vi "Control Experiment.vi"() -> ()   [LabVIEW 2016, in "Transport.lvclass"]
uses:
  Transport.lvclass
  <userlib>/LevyLab/Krohn Hite 7008/typedefs/Shunt-Enum.ctl
  <userlib>/LevyLab/Krohn Hite 7008/typedefs/Gain-Enum.ctl
  <userlib>/LevyLab/Krohn Hite 7008/typedefs/KH_control_array.ctl
  <userlib>/LevyLab/Krohn Hite 7008/typedefs/KH_control.ctl
  <userlib>/LevyLab/Krohn Hite 7008/typedefs/Channel-Enum.ctl
  <userlib>/LevyLab/Krohn Hite 7008/typedefs/Input Configuration-Enum.ctl
  levylab_inst_pickering/lvsrc/SMOs/pickering/Typedefs/PickeringConfig-Cluster.ctl
  levylab_inst_pickering/lvsrc/SMOs/pickering/Typedefs/PickeringXConfig-Cluster.ctl
  levylab_inst_pickering/lvsrc/SMOs/pickering/Typedefs/PickeringYConfig-Cluster.ctl
  Control Experiment FGV-cluster.ctl
  ITX_Global.vi
  Channel Global.vi
  <userlib>/LevyLab/Krohn Hite 7008/KH7008.lvclass
  <vilib>/addons/_JKI.lib/Serialization/JSON/JKI JSON Serialization.lvlib
  levylab_inst_pickering/lvsrc/SMOs/pickering/pickering.lvclass
panel:
  in  "Create Output":bool
  in  "OK":bool
  in  "Tab Control":T1(tab)=enum."Pickering Configuration"
  in  "Pickering Buttons":enum32{"Pickering", "Not Pickering"}(radio)
  in  "description":string="graphene"
  in  "KH Configuration":enum16{"Ground", "Current", "Voltage", "Gate"}[](array[ring])=[enum."Current", enum."Current", enum."Ground", enum."Ground", enum."Ground", enum."Ground", enum."Ground", enum."Ground"]
  in  "KH Shunt Resistor":T2[](array[typedef])=[enum."50 Ohms", enum."50 Ohms", enum."50 Ohms", enum."50 Ohms", enum."50 Ohms", enum."50 Ohms", enum."50 Ohms", enum."50 Ohms"]
  in  "KH Gain":T3[](array[typedef])=[enum."10x", enum."10x", enum."10x", enum."10x", enum."10x", enum."10x", enum."10x", enum."10x"]
  in  "KH Ch":enum16{"1", "2", "3", "4", "5", "6", "7", "8"}[](array[ring])=[enum."1", enum."2", enum."3", enum."4", enum."5", enum."6", enum."7", enum."8"]
  in  "Electrode":T4(array[ring])=[enum."26", enum."26", enum."NC", enum."NC", enum."NC", enum."NC", enum."NC", enum."NC"]
  in  "Lockin Ch":enum16{"1", "2", "3", "4", "5", "6", "7", "8"}[](array[ring])=[enum."1", enum."2", enum."3", enum."4", enum."5", enum."6", enum."7", enum."8"]
  in  "Label":u16[](array[ring]) items=["", "I+", "I-", "V1+", "V1-", "V2+", "V2-", "V3+", "V3-", "V4+", "V4-", "Vsg", "Vbg"]
  in  "sample":string="SA01234"
  in  "device 2":string="20180713"
  in  "project (enum?)":string="graphene"
  in  "user (emum?)":string="patrick"
  in  "canvas":string="SA01234"
  in  "KH ALL Buttons":T5(radio)
  in  "Write Pickering Config":bool
  in  "Labels":u16[](array[ring]) items=["", "I+", "I-", "V1+", "V1-", "V2+", "V2-", "V3+", "V3-", "V4+", "V4-", "Vsg", "Vbg"]
  in  "Electrodes":T4(array[ring])
  in  "Y Channels":string[][](array[combo])=[["y1", "NC"], ["y2", "NC"], ["y3", ""], ["y4", ""], ["y5", ""], ["y6", ""], ["y7", ""], ["y8", ""], ["NC", ""], ["y7", ""], ["y6", ""]]
  in  "X Channels":string[](array[combo])=["x1", "x2", "x3", "x4", "x5", "x6", "x7", "x8", "x9", "x10", "x11", "x12"]
  out "X Channel Array":string[](array[string])
  out "Y Channel Array":string[][](array[string])
  in  "Read Pickering Config":bool
  out "device":string="SA01234SA01234.20180713"
  out "comments":string="SA01234SA01234.20180713\rgraphene\rpatrick\r2018-08-29T14:08:0929\r\rLockin1: 26\tI+\rLockin2: 26\tI-\rLockin3: NC\tV4-\rLockin4: NC\tV2+\rLockin5: NC\tV3+\rLockin6: NC\tV2-\rLockin7: NC\tV1+\rLockin8: NC\tV4+\r\n"
  out "folder":string="G:\\Team Drives\\LevyLabData\\graphene\\SA01234SA01234.20180713"
  out "filename":string="SA01234SA01234.20180713"
  out "JSON String":string="{\r\n    \"sample\":\"SA01234\",\r\n    \"canvas\":\"SA01234\",\r\n    \"date\":\"20180713\",\r\n    \"user\":\"patrick\",\r\n    \"project\":\"graphene\",\r\n    \"path\":\"G:\\\\Team Drives\\\\LevyLabData\\\\graphene\\\\SA01234SA01234.20180713\",\r\n    \"device\":\"SA01234SA01234.20180713\",\r\n    \"Channel Setting\":[\r\n        {\r\n            \"Channel\":\"Channel 1\",\r\n            \"Gain\":\"10x\",\r\n            \"Shunt Resistor\":\"50 Ohms\",\r\n            \"Input Config\":\"Differential\"\r\n        },\r\n        {\r\n            \"Channel\":\"Channel 2\",\r\n            \"Gain\":\"10x\",\r\n            \"Shunt Resistor\":\"50 Ohms\",\r\n            \"Input Config\":\"Differential\"\r\n        },\r\n        {\r\n            \"Channel\":\"Channel 3\",\r\n            \"Gain\":\"1x\",\r\n            \"Shunt Resistor\":\"Open\",\r\n            \"Input Config\":\"Ground\"\r\n        },\r\n        {\r\n            \"Channel\":\"Channel 4\",\r\n            \"Gain\":\"1x\",\r\n            \"Shunt Resistor\":\"Open\",\r\n            \"Input Config\":\"Ground\"\r\n        },\r\n        {\r\n            \"Channel\":\"Channel 5\",\r\n            \"Gain\":\"1x\",\r\n            \"Shunt Resistor\":\"Open\",\r\n            \"Input Config\":\"Ground\"\r\n        },\r\n        {\r\n            \"Channel\":\"Channel 6\",\r\n            \"Gain\":\"1x\",\r\n            \"Shunt Resistor\":\"Open\",\r\n            \"Input Config\":\"Ground\"\r\n        },\r\n        {\r\n            \"Channel\":\"Channel 7\",\r\n            \"Gain\":\"1x\",\r\n            \"Shunt Resistor\":\"Open\",\r\n            \"Input Config\":\"Ground\"\r\n        },\r\n        {\r\n            \"Channel\":\"Channel 8\",\r\n            \"Gain\":\"1x\",\r\n            \"Shunt Resistor\":\"Open\",\r\n            \"Input Config\":\"Ground\"\r\n        }\r\n    ],\r\n    \"All same as ch1?\":false,\r\n    \"Lockin Ch\":[\r\n        \"1\",\r\n        \"2\",\r\n        \"3\",\r\n        \"4\",\r\n        \"5\",\r\n        \"6\",\r\n        \"7\",\r\n        \"8\"\r\n    ],\r\n    \"KH Ch\":[\r\n        \"1\",\r\n        \"2\",\r\n        \"3\",\r\n        \"4\",\r\n        \"5\",\r\n        \"6\",\r\n        \"7\",\r\n        \"8\"\r\n    ],\r\n    \"Gain\":[\r\n        \"10x\",\r\n        \"10x\",\r\n        \"10x\",\r\n        \"10x\",\r\n        \"10x\",\r\n        \"10x\",\r\n        \"10x\",\r\n        \"10x\"\r\n    ],\r\n    \"Configuration\":[\r\n        \"Current\",\r\n        \"Current\",\r\n        \"Ground\",\r\n        \"Ground\",\r\n        \"Ground\",\r\n        \"Ground\",\r\n        \"Ground\",\r\n        \"Ground\"\r\n    ],\r\n    \"Shunt Resistor\":[\r\n        \"50 Ohms\",\r\n        \"50 Ohms\",\r\n        \"50 Ohms\",\r\n        \"50 Ohms\",\r\n        \"50 Ohms\",\r\n        \"50 Ohms\",\r\n        \"50 Ohms\",\r\n        \"50 Ohms\"\r\n    ],\r\n    \"Electrode\":[\r\n        \"26\",\r\n        \"26\",\r\n        \"NC\",\r\n        \"NC\",\r\n        \"NC\",\r\n        \"NC\",\r\n        \"NC\",\r\n        \"NC\"\r\n    ],\r\n    \"Label\":[\r\n        \"I+\",\r\n        \"I-\",\r\n        \"V4-\",\r\n        \"V2+\",\r\n        \"V3+\",\r\n        \"V2-\",\r\n        \"V1+\",\r\n        \"V4+\"\r\n    ]\r\n}"
  in  "Strings []":string[](array[string])
  in  "Enum":T6(ring)=enum."V2-"
  out "YAML example":string="description: This is a dummy dataset which mimics smFRET data.\n\nsetup:\n    ## Mandatory fields\n    num_pixels: 2                # using 2 detectors\n    num_spots: 1                 # a single confocal excitation\n    num_spectral_ch: 2           # donor and acceptor detection\n    num_polarization_ch: 1       # no polarization selection\n    num_split_ch: 1              # no beam splitter\n    modulated_excitation: False  # CW excitation, no modulation\n    lifetime: False              # no TCSPC in detection\n\n    ## Optional fields\n    excitation_wavelengths:      # List of excitation wavelenghts\n       - !!float 532e-9\n    excitation_cw:               # List of booleans, True if wavelength is CW\n       - True\n    detection_wavelengths:       # Nominal center wavelength for each for detection ch\n       - !!float 580e-9\n       - !!float 640e-9\n\nsample:\n  sample_name: describe the sample here\n  buffer_name: describe the buffer here\n  dye_names: 'Cy3B, ATTO647N'   # Comma separates names of fluorophores\n\nidentity:\n    author: Author Name\n    author_affiliation: Name of Research Institution\n\nprovenance:\n    filename: 'photon_data.hdf5'\n    software: Acquisition Software Name\n\nphoton_data:\n    timestamps_specs:\n        timestamps_unit: !!float 10e-9  # 10 ns\n    measurement_specs:\n        measurement_type: smFRET\n        detectors_specs:\n            spectral_ch1: [0]  # list of donor's detector IDs\n            spectral_ch2: [1]  # list of acceptor's detector IDs"
  # "1. need a way to associate lockin channels with arbitrary KH  channels (e.g. lockin 1\nis connected to 7. Lockin needs to read appropriate gain from KH)\n2. All grounded or all differential button for KH  is good\n3. add additional notes?"
  # "how to enforce unique choice of label?"
  # "some of these are used to set KH\nsome are just saved as meta data\nsome are used"
  # "how to sell?\nshow what it is replacing\n(KH control, Channel Globals, Lockin 0 vs 1 nonsene, typing into comments)"
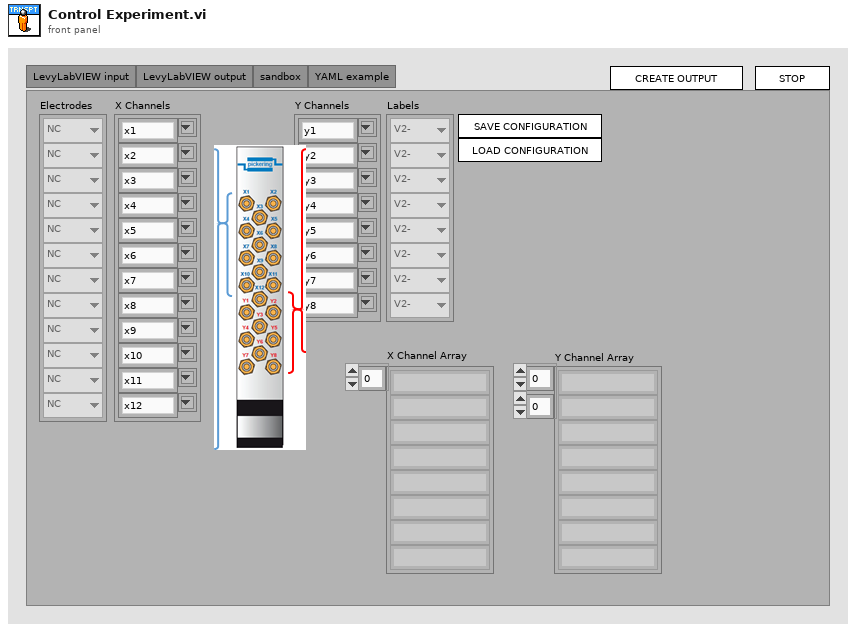
[diagram p1: front panel]
types:
  T1 = enum32{"LevyLabVIEW input", "Pickering Configuration", "LevyLabVIEW output", "sandbox", "YAML example"}
  T2 = typedef "KH7008.lvclass/Shunt-Enum.ctl" = enum16{"Open", "50 Ohms", "500 Ohms", "5k Ohms", "50k Ohms"}
  T3 = typedef "KH7008.lvclass/Gain-Enum.ctl" = enum16{"1x", "10x", "100x", "1000x"}
  T4 = enum16{"NC", "26", "27", "28", "1", "2", "3", "4", "5", "6", "7", "8", "9", "10", "11", "12", "13", "14", "15", "16", "17", "18", "19", "20", "21", "22", "23", "24", "25"}[]
  T5 = enum32{"No Selection", "all ground", "all differential"}
  T6 = enum16{"", "I+", "I-", "V1+", "V1-", "V2+", "V2-", "V3+", "V3-", "V4+", "V4-", "Vsg", "Vbg"}
  T7 = enum8{"Enabled", "Disabled", "Disabled and Grayed Out"}
  T8 = enum32{"invalid app kind", "Development System", "Run Time System", "Student Edition", "Embedded LabVIEW", "Evaluation", "Custom"}
  T9 = enum32{"Invalid", "Standard", "Closed", "Hidden", "Minimized", "Maximized"}
  T10 = typedef "KH7008.lvclass/Input Configuration-Enum.ctl" = enum16{"Ground", "SE+ (-gnd)", "SE- (+gnd)", "Differential"}
  T11 = typedef "pickering.lvclass/PickeringConfig-Cluster.ctl" = cluster{"x config":T12, "y config":T13}
  T12 = typedef "pickering.lvclass/PickeringXConfig-Cluster.ctl" = cluster{"Electrode":enum16{"NC", "26", "27", "28", "1", "2", "3", "4", "5", "6", "7", "8", "9", "10", "11", "12", "13", "14", "15", "16", "17", "18", "19", "20", "21", "22", "23", "24", "25"}[], "X Channels":string[]}
  T13 = typedef "pickering.lvclass/PickeringYConfig-Cluster.ctl" = cluster{"Label":u16[], "Y Channels":string[][]}
  T14 = typedef "Transport.lvclass/Control Experiment FGV-cluster.ctl" = cluster{"path":path, "device":string, "user":string, "comments":string, "Lockin Ch":enum16{"1", "2", "3", "4", "5", "6", "7", "8"}[], "Electrode":enum16{"NC", "26", "27", "28", "1", "2", "3", "4", "5", "6", "7", "8", "9", "10", "11", "12", "13", "14", "15", "16", "17", "18", "19", "20", "21", "22", "23", "24", "25"}[], "Label":u16[], "KH Ch":enum16{"1", "2", "3", "4", "5", "6", "7", "8"}[], "Configuration":enum16{"Ground", "Current", "Voltage", "Gate"}[], "Gain":T3[], "Shunt Resistor":T2[]}
  T15 = typedef "KH7008.lvclass/KH_control_array.ctl" = T16[]
  T16 = typedef "KH7008.lvclass/KH_control.ctl" = cluster{"Channel":T17, "Gain":T3, "Shunt Resistor":T2, "Input Config":T10}
  T17 = typedef "KH7008.lvclass/Channel-Enum.ctl" = enum16{"Channel 1", "Channel 2", "Channel 3", "Channel 4", "Channel 5", "Channel 6", "Channel 7", "Channel 8"}
  T18 = cluster{"Core":cluster{"Current VI Reference":refnum<vi>, "Close Panel on Exit?":bool}, "sample":string, "canvas":string, "date":string, "user":string, "project":string, "path":path, "device":string, "Channel Setting":T15, "KH ALL Buttons":enum32{"No Selection", "all ground", "all differential"}, "Lockin Ch":enum16{"1", "2", "3", "4", "5", "6", "7", "8"}[], "KH Ch":enum16{"1", "2", "3", "4", "5", "6", "7", "8"}[], "Gain":T3[], "Configuration":enum16{"Ground", "Current", "Voltage", "Gate"}[], "Shunt Resistor":T2[], "Electrode":enum16{"NC", "26", "27", "28", "1", "2", "3", "4", "5", "6", "7", "8", "9", "10", "11", "12", "13", "14", "15", "16", "17", "18", "19", "20", "21", "22", "23", "24", "25"}[], "Label":u16[], "comments":string}
  T19 = cluster{"Current VI Reference":refnum<vi>, "Close Panel on Exit?":bool}
  T20 = cluster{"description":string, "device":string, "project":string, "user":string, "Lockin Ch":enum16{"1", "2", "3", "4", "5", "6", "7", "8"}[], "KH Ch":enum16{"1", "2", "3", "4", "5", "6", "7", "8"}[], "Gain":T3[], "Configuration":enum16{"Ground", "Current", "Voltage", "Gate"}[], "Shunt Resistor":T2[], "Electrode":enum16{"NC", "26", "27", "28", "1", "2", "3", "4", "5", "6", "7", "8", "9", "10", "11", "12", "13", "14", "15", "16", "17", "18", "19", "20", "21", "22", "23", "24", "25"}[], "Label":u16[]}
  T21 = cluster{"sample":string, "canvas":string, "date":string, "user":string, "project":string, "path":path, "device":string, "Channel Setting":T15, "KH ALL Buttons":enum32{"No Selection", "all ground", "all differential"}, "Lockin Ch":enum16{"1", "2", "3", "4", "5", "6", "7", "8"}[], "KH Ch":enum16{"1", "2", "3", "4", "5", "6", "7", "8"}[], "Gain":T3[], "Configuration":enum16{"Ground", "Current", "Voltage", "Gate"}[], "Shunt Resistor":T2[], "Electrode":enum16{"NC", "26", "27", "28", "1", "2", "3", "4", "5", "6", "7", "8", "9", "10", "11", "12", "13", "14", "15", "16", "17", "18", "19", "20", "21", "22", "23", "24", "25"}[], "Label":u16[]}
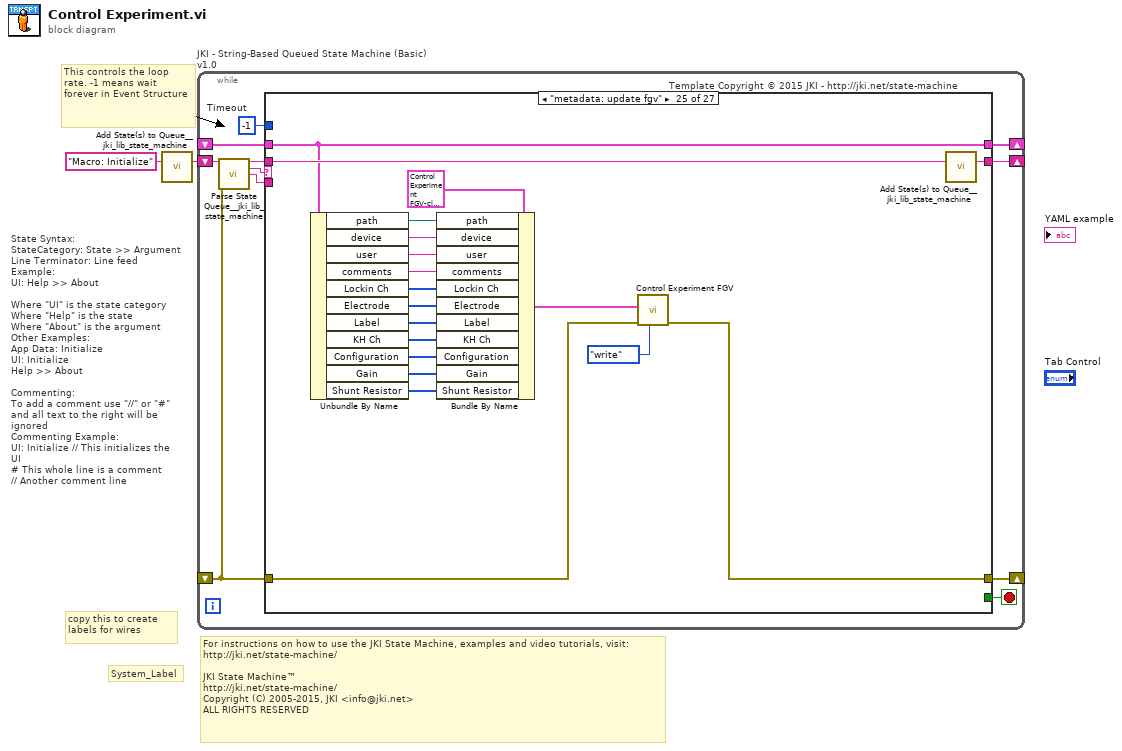
[diagram p0: block diagram]
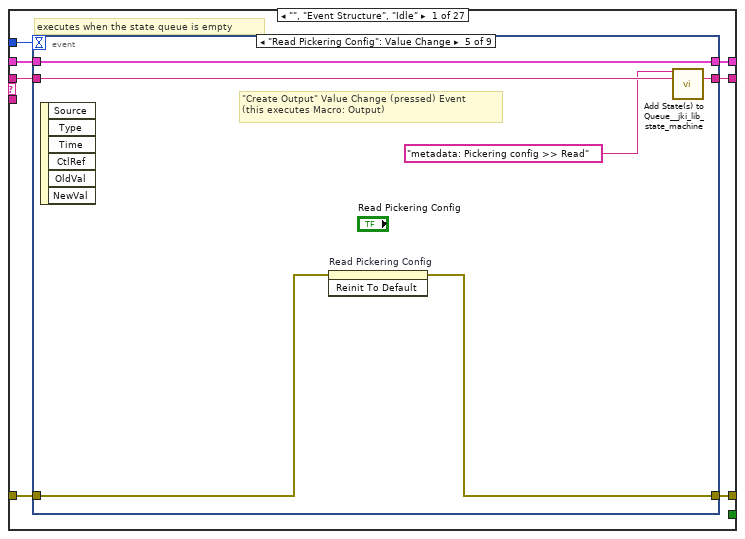
[diagram p2: hidden frame]
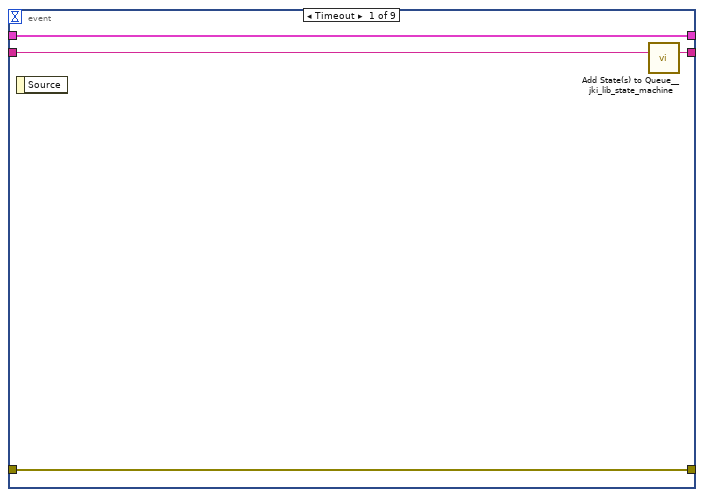
[diagram p3: hidden frame]
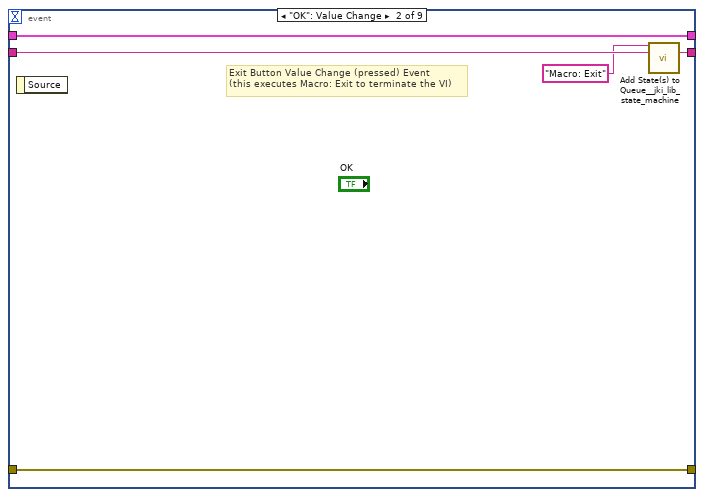
[diagram p4: hidden frame]
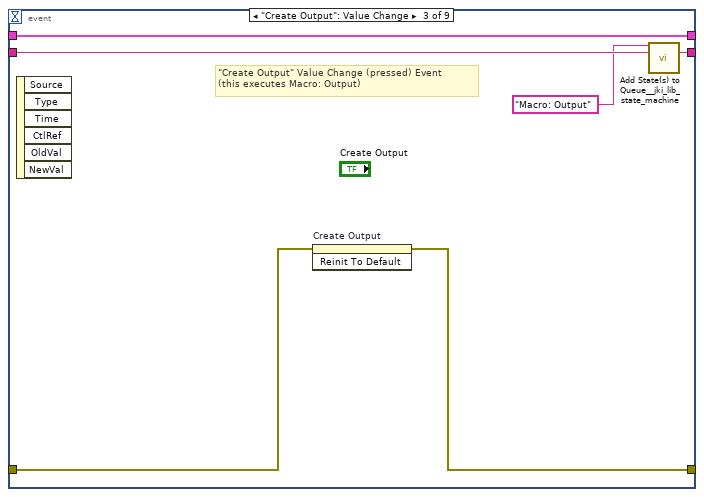
[diagram p5: hidden frame]
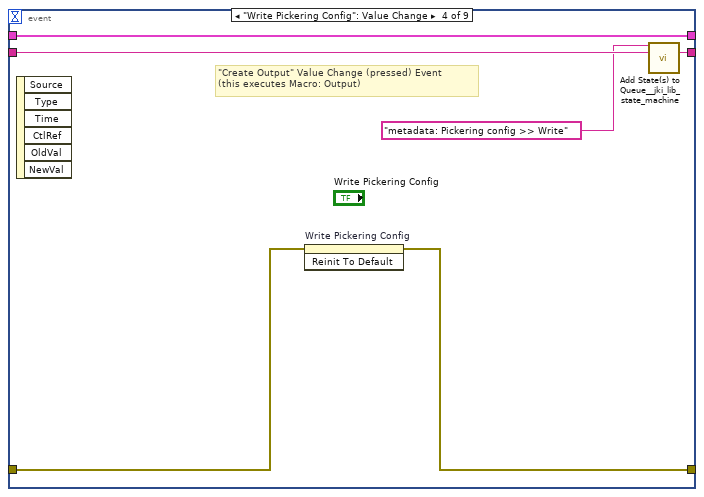
[diagram p6: hidden frame]
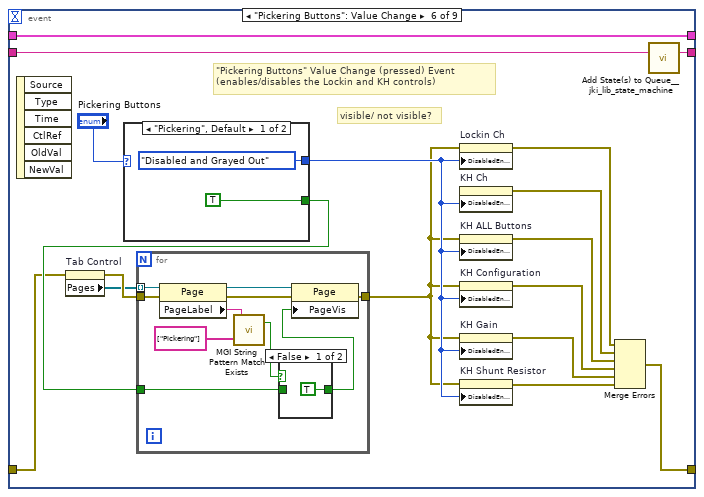
[diagram p7: hidden frame]
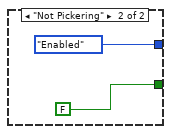
[diagram p9: hidden frame]
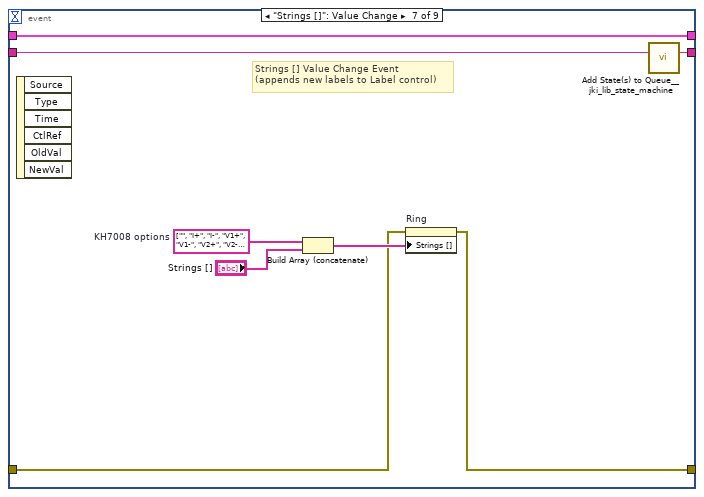
[diagram p10: hidden frame]
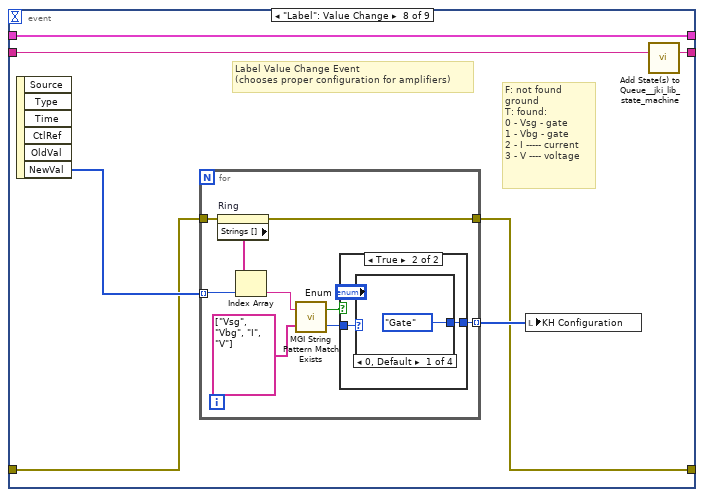
[diagram p11: hidden frame]
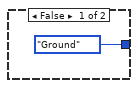
[diagram p12: hidden frame]
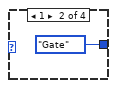
[diagram p13: hidden frame]
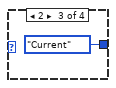
[diagram p14: hidden frame]
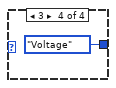
[diagram p15: hidden frame]
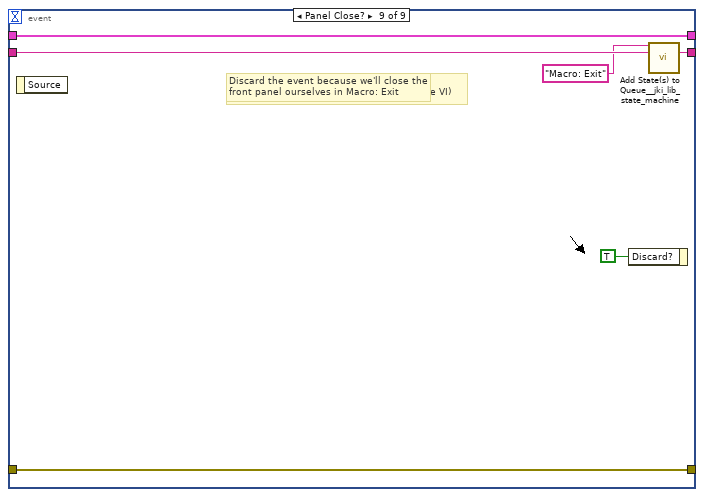
[diagram p16: hidden frame]
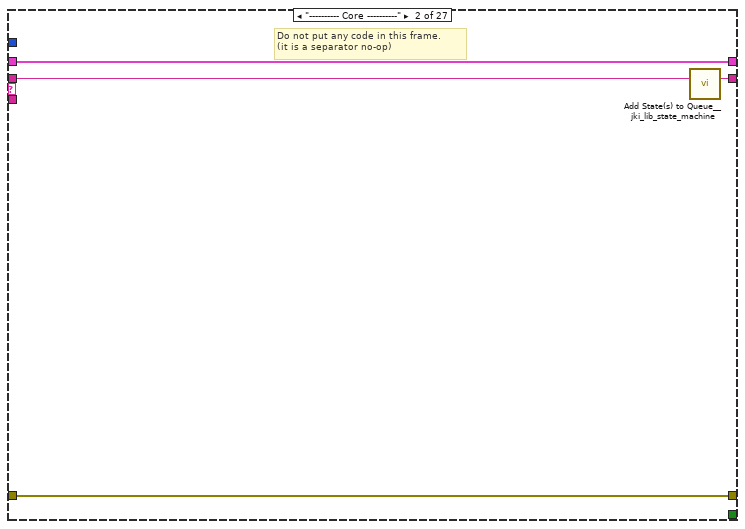
[diagram p17: hidden frame]
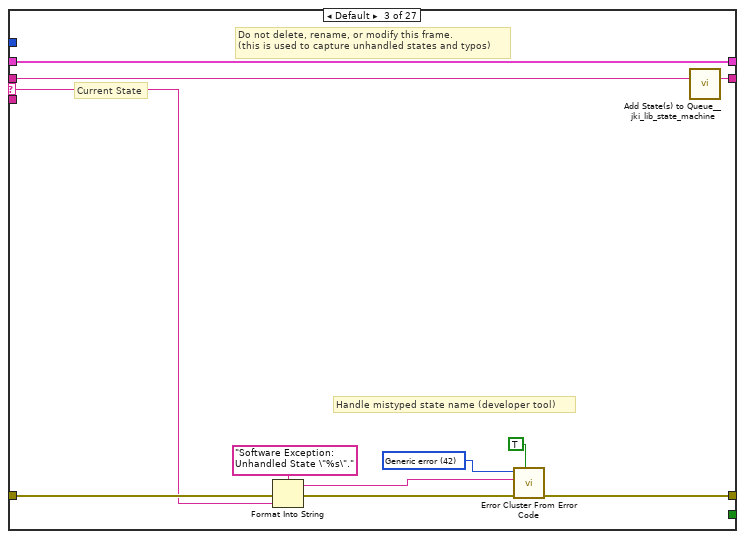
[diagram p18: hidden frame]
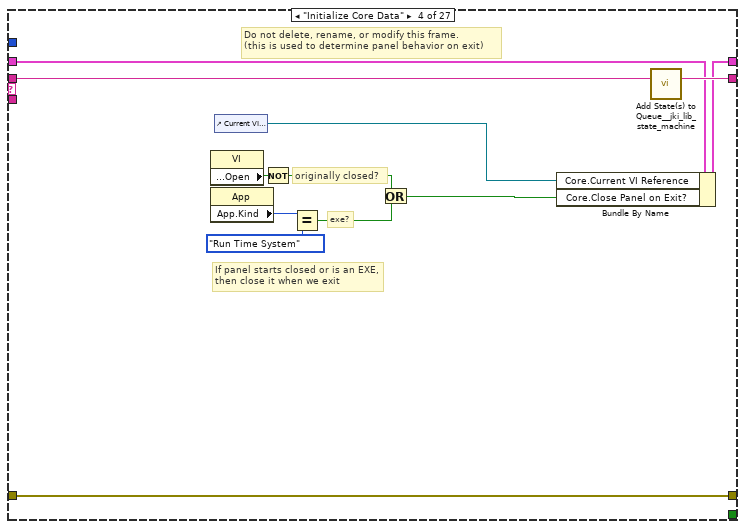
[diagram p19: hidden frame]
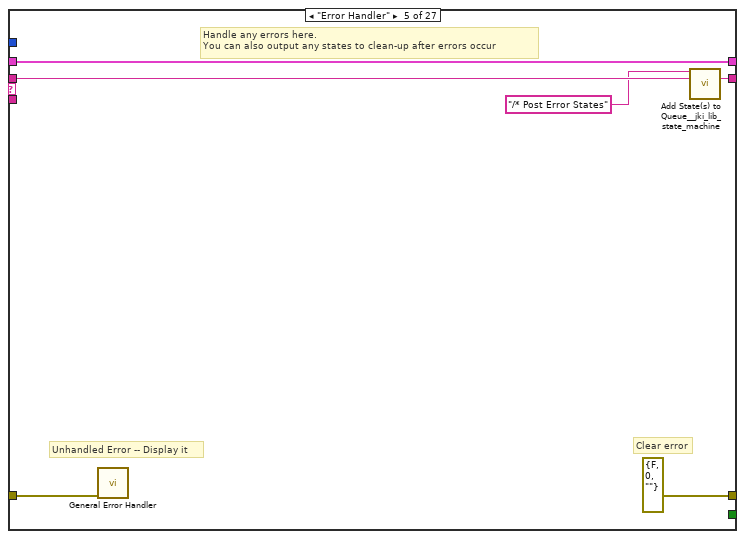
[diagram p20: hidden frame]
diagram:
  # "For instructions on how to use the JKI State Machine, examples and video tutorials, visit:\nhttp://jki.net/state-machine/\n\nJKI State Machine™\nhttp://jki.net/state-machine/\nCopyright (C) 2005-2015, JKI <info@jki.net>\nALL RIGHTS RESERVED"
  # "State Syntax:\nStateCategory: State >> Argument\nLine Terminator: Line feed\nExample:\nUI: Help >> About\n\nWhere \"UI\" is the state category\nWhere \"Help\" is the state\nWhere \"About\" is the argument\nOther Examples:\nApp Data: Initialize\nUI: Initialize\nHelp >> About\n\nCommenting:\nTo add a comment use \"//\" or \"#\" and all text to the right will be ignored\nCommenting Example:\nUI: Initialize // This initializes the UI\n# This whole line is a comment\n// Another comment line"
  # "copy this to create labels for wires"
  # "This controls the loop rate. -1 means wait forever in Event Structure"
  # "System_Label"
  n1 = call <vilib>:"Add State(s) to Queue__jki_lib_state_machine.vi"("State(s) in (\"\")"="Macro: Initialize") -> ("States Out"=w2:string)  [unwired: 14 in]
  n2 = while "JKI - String-Based Queued State Machine (Basic) v1.0" {
    shift-right: [w6] -> _
    shift-left: _ -> [w5]
    shift-right: [w9] -> _
    shift-left: _ -> [w3]
    shift-right: [w8] -> _
    shift-left: w2 -> [w10]
    stop <- w7 stop-if-true
    w4 = -1  # Timeout
    # "Template Copyright © 2015 JKI - http://jki.net/state-machine"
    n3 = call <vilib>:"Parse State Queue__jki_lib_state_machine.vi"("State Queue"=w10, "Error In (no error)"=w3) -> ("Remaining States"=w12:string, "Current State"=w13:string, "Arguments"=w11:string)  [unwired: 11 in]
    n4 = case shown="\"metadata: update fgv\"" w13 {
      selector: w13 -> [_ _ w122 _ _ _ _ _ _ _ _ _ _ _ _ _ _ _ _ _ _ _ _ _ _ _ _]
      tunnel: w12 -> [w20 w121 w126 w144 w150 w155 w159 w181 w187 w191 w201 w207 w218 w244 w249 w259 w268 w274 w293 w311 w349 w359 w387 w395 w451 w470 w495]
      tunnel: w11 -> [_ _ _ _ _ _ _ _ _ _ _ w202 w212 _ _ _ _ _ _ _ _ w354 _ _ _ _ _]
      tunnel: w5 -> [w18 w118 w124 w135 w147 w153 w156 _ w182 w188 w199 w205 w214 w241 w246 w256 w265 w271 w290 w301 w347 w357 w382 w390 w449 w453 w488]
      tunnel: [w17 w119 w128 w141 errorcluster {"status"=FALSE, "code"=0, "source"=""} ("error out") w152 w157 w178 w183 w189 w194 w203 w215 w242 w247 w257 w266 w272 w291 w303 w346 w355 w385 w393 w435 w468 w489] -> w9
      tunnel: w3 -> [w16 w119 w127 w141 w146 w152 w157 w178 w184 w189 w198 w204 w216 w242 w247 w257 w266 w272 w291 w304 w343 w356 w385 w393 w436 w455 w490]
      tunnel: [w19 w120 w125 w143 w149 w154 w158 w180 w186 w190 w200 w206 w217 w243 w248 w258 w267 w273 w292 w310 w348 w358 w386 w394 w450 w469 w494] -> w8
      tunnel: [_ _ _ _ _ TRUE _ _ _ _ _ _ _ _ _ _ _ _ _ _ _ _ _ _ _ _ _] -> w7
      tunnel: [w15 w118 w124 w142 w147 w153 w156 w179 w182 w188 w199 w205 w214 w241 w246 w256 w265 w271 w289 w300 w347 w357 w381 w390 w449 w453 w488] -> w6
      tunnel: w4 -> [w14 _ _ _ _ _ _ _ _ _ _ _ _ _ _ _ _ _ _ _ _ _ _ _ _ _ _]
      frame "", "Event Structure", "Idle" {
        # "executes when the state queue is empty"
        n5 = event shown="[4] \"Read Pickering Config\": Value Change" {
          selector: _ -> [_ _ _ _ _ _ _ _ _]
          dyn-events: _ -> [_ _ _ _ _ _ _ _ _]
          timeout: w14 -> [_ _ _ _ _ _ _ _ _]
          tunnel: w20 -> [w24 w29 w35 w41 w47 w64 w88 w95 w117]
          tunnel: [w23 w28 w34 w40 w46 w63 w87 w94 w116] -> w19
          tunnel: w18 -> [w21 w26 w33 w39 w45 w62 w86 w93 w114]
          tunnel: [w22 w27 w30 w36 w42 w54 w83 w89 w115] -> w17
          tunnel: w16 -> [w22 w27 w31 w37 w43 w50 w84 w90 w115]
          tunnel: [w21 w26 w33 w39 w45 w62 w86 w93 w114] -> w15
          event Timeout {
            n6 = event-data() -> ()  [unwired: 1 in, 1 out]
            n7 = call <vilib>:"Add State(s) to Queue__jki_lib_state_machine.vi"("State(s) in (\"\")"=w24) -> ("States Out"=w23:string)  [unwired: 14 in]
          }
          event "OK": Value Change {
            # "Exit Button Value Change (pressed) Event\n(this executes Macro: Exit to terminate the VI)"
            n8 = event-data() -> ()  [unwired: 1 in, 1 out]
            n9 = call <vilib>:"Add State(s) to Queue__jki_lib_state_machine.vi"("State(s) in Front (\"\")"="Macro: Exit", "State(s) in (\"\")"=w29) -> ("States Out"=w28:string)  [unwired: 13 in]
          }
          event "Create Output": Value Change {
            # "\"Create Output\" Value Change (pressed) Event\n(this executes Macro: Output)"
            n10 = event-data() -> ()  [unwired: 1 in, 6 out]
            n11 = invoke on="Create Output" class="Bool" method="Reinit To Default"(error in=w31) -> (error out=w30:errorcluster)  [unwired: 2 in, 2 out]
            n12 = call <vilib>:"Add State(s) to Queue__jki_lib_state_machine.vi"("State(s) in Front (\"\")"="Macro: Output", "State(s) in (\"\")"=w35) -> ("States Out"=w34:string)  [unwired: 13 in]
          }
          event "Write Pickering Config": Value Change {
            # "\"Create Output\" Value Change (pressed) Event\n(this executes Macro: Output)"
            n13 = event-data() -> ()  [unwired: 1 in, 6 out]
            n14 = invoke on="Write Pickering Config" class="Bool" method="Reinit To Default"(error in=w37) -> (error out=w36:errorcluster)  [unwired: 2 in, 2 out]
            n15 = call <vilib>:"Add State(s) to Queue__jki_lib_state_machine.vi"("State(s) in Front (\"\")"="metadata: Pickering config >> Write", "State(s) in (\"\")"=w41) -> ("States Out"=w40:string)  [unwired: 13 in]
          }
          event "Read Pickering Config": Value Change {
            # "\"Create Output\" Value Change (pressed) Event\n(this executes Macro: Output)"
            n16 = event-data() -> ()  [unwired: 1 in, 6 out]
            n17 = invoke on="Read Pickering Config" class="Bool" method="Reinit To Default"(error in=w43) -> (error out=w42:errorcluster)  [unwired: 2 in, 2 out]
            n18 = call <vilib>:"Add State(s) to Queue__jki_lib_state_machine.vi"("State(s) in Front (\"\")"="metadata: Pickering config >> Read", "State(s) in (\"\")"=w47) -> ("States Out"=w46:string)  [unwired: 13 in]
          }
          event "Pickering Buttons": Value Change {
            # "visible/ not visible?"
            # "\"Pickering Buttons\" Value Change (pressed) Event\n(enables/disables the Lockin and KH controls)"
            n19 = event-data() -> ()  [unwired: 1 in, 6 out]
            n20 = property on="Tab Control" class="TabCtl (strict)"(error in=w50) -> (error out=w53:errorcluster, "Pages"=w52:refnum<vi>[])  [unwired: 1 in, 1 out]
            n21 = case shown="\"Pickering\", Default" "Pickering Buttons" {
              tunnel: [T7."Disabled and Grayed Out" ("Disabled") T7."Enabled" ("Disabled")] -> w61
              tunnel: [TRUE ("Page Visible") FALSE ("Page Visible")] -> w51
              frame "Pickering", Default {
              }
              frame "Not Pickering" {
              }
            }
            n22 = for {
              tunnel: w52 -> [w74] mode=indexing
              tunnel: w53 -> [w70]
              tunnel: w51 -> [w68]
              tunnel: [w67] -> w49
              n23 = property class="Page"(reference=w74, error in=w70) -> (reference out=w71:refnum<vi>, error out=w69:errorcluster, "PageLabel"=w73:string)
              n24 = call <userlib>:"MGI String Pattern Match Exists.vi"("Patterns to Try"=string[] ["Pickering"], "String"=w73) -> ("Match Found"=w66:bool)  [unwired: 1 out]
              n25 = case shown="False" w66 {
                tunnel: [TRUE ("Page Visible") w76] -> w65
                tunnel: w68 -> [_ w76]
                frame False {
                }
                frame True {
                }
              }
              n26 = property class="Page"(reference=w71, error in=w69, "PageVis"=w65) -> (error out=w67:errorcluster)  [unwired: 1 out]
            }
            n27 = property on="Lockin Ch" class="Arr (strict)"(error in=w49, "DisabledEnum"=w61) -> (error out=w55:errorcluster)  [unwired: 1 in, 1 out]
            n28 = property on="KH Ch" class="Arr (strict)"("DisabledEnum"=w61) -> (error out=w56:errorcluster)  [unwired: 2 in, 1 out]
            n29 = property on="KH ALL Buttons" class="RadioBtnsControl (strict)"(error in=w49, "DisabledEnum"=w61) -> (error out=w57:errorcluster)  [unwired: 1 in, 1 out]
            n30 = property on="KH Configuration" class="Arr (strict)"(error in=w49, "DisabledEnum"=w61) -> (error out=w58:errorcluster)  [unwired: 1 in, 1 out]
            n31 = property on="KH Gain" class="Arr (strict)"(error in=w49, "DisabledEnum"=w61) -> (error out=w59:errorcluster)  [unwired: 1 in, 1 out]
            n32 = property on="KH Shunt Resistor" class="Arr (strict)"(error in=w49, "DisabledEnum"=w61) -> (error out=w60:errorcluster)  [unwired: 1 in, 1 out]
            n33 = Merge Errors(w55, w56, w57, w58, w59, w60) -> (w54:errorcluster)
            n34 = call <vilib>:"Add State(s) to Queue__jki_lib_state_machine.vi"("State(s) in (\"\")"=w64) -> ("States Out"=w63:string)  [unwired: 14 in]
          }
          event "Strings []": Value Change {
            w81 = string[] ["", "I+", "I-", "V1+", "V1-", "V2+", "V2-", "V3+", "V3-", "V4+", "V4-", "Vsg"]  # KH7008 options
            # "Strings [] Value Change Event\n(appends new labels to Label control)"
            n35 = event-data() -> ()  [unwired: 1 in, 6 out]
            n36 = Build Array (concatenate)(w81, "Strings []") -> (w85:string[])
            n37 = property on="Ring" class="Ring (strict)"(error in=w84, "Strings []"=w85) -> (error out=w83:errorcluster)  [unwired: 1 in, 1 out]
            n38 = call <vilib>:"Add State(s) to Queue__jki_lib_state_machine.vi"("State(s) in (\"\")"=w88) -> ("States Out"=w87:string)  [unwired: 14 in]
          }
          event "Label": Value Change {
            # "F: not found\nground\nT: found:\n0 - Vsg - gate\n1 - Vbg - gate\n2 - I ----- current\n3 - V ---- voltage"
            # "Label Value Change Event\n(chooses proper configuration for amplifiers)"
            n39 = event-data() -> ("NewVal"=w92:u16[])  [unwired: 1 in, 5 out]
            n40 = for {
              tunnel: w92 -> [w100] mode=indexing
              tunnel: [w102] -> w91 mode=indexing
              tunnel: w90 -> [w99]
              tunnel: [w98] -> w89
              n41 = property on="Ring" class="Ring (strict)"(error in=w99) -> (error out=w98:errorcluster, "Strings []"=w101:string[])  [unwired: 1 in, 1 out]
              n42 = Index Array(array=w101, index=w100) -> (element=w97:string)
              n43 = call <userlib>:"MGI String Pattern Match Exists.vi"("Patterns to Try"=string[] ["Vsg", "Vbg", "I", "V"], "String"=w97) -> ("Index of First Pattern Matched"=w103:i32, "Match Found"=w104:bool)
              n44 = case shown="True" w104 {
                tunnel: w103 -> [_ w107]
                tunnel: [enum16{"Ground", "Current", "Voltage", "Gate"}."Ground" ("Enum") w106] -> w102
                frame False {
                }
                frame True {
                  n45 = case shown="0, Default" w107 {
                    tunnel: [enum16{"Ground", "Current", "Voltage", "Gate"}."Gate" ("Enum") enum16{"Ground", "Current", "Voltage", "Gate"}."Gate" ("Enum") enum16{"Ground", "Current", "Voltage", "Gate"}."Current" ("Enum") enum16{"Ground", "Current", "Voltage", "Gate"}."Voltage" ("Enum")] -> w106
                    frame 0, Default {
                    }
                    frame 1 {
                    }
                    frame 2 {
                    }
                    frame 3 {
                    }
                  }
                }
              }
            }
            n46 = local write "KH Configuration"(w91) -> ()
            n47 = call <vilib>:"Add State(s) to Queue__jki_lib_state_machine.vi"("State(s) in (\"\")"=w95) -> ("States Out"=w94:string)  [unwired: 14 in]
          }
          event Panel Close? {
            # "Discard the event because we'll close the front panel ourselves in Macro: Exit"
            # "Close Panel button (pressed) Event\n(this executes Macro: Exit to terminate the VI)"
            n48 = event-data() -> ()  [unwired: 1 in, 1 out]
            n49 = event-data("Discard?"=TRUE) -> ()  [unwired: 1 in, 1 out]
            n50 = call <vilib>:"Add State(s) to Queue__jki_lib_state_machine.vi"("State(s) in Front (\"\")"="Macro: Exit", "State(s) in (\"\")"=w117) -> ("States Out"=w116:string)  [unwired: 13 in]
          }
        }
      }
      frame "---------- Core ----------" {
        # "Do not put any code in this frame.\n(it is a separator no-op)"
        n51 = call <vilib>:"Add State(s) to Queue__jki_lib_state_machine.vi"("State(s) in (\"\")"=w121) -> ("States Out"=w120:string)  [unwired: 14 in]
      }
      frame Default {
        w131 = 42 items=["No error", "Argument error", "Memory is full", "Out of zone", "End of file", "File already open", "Generic file I/O error", "File not found", "File permission error", "Disk is full", "Duplicate path", "Too many files open", "System feature not enabled", "Resource file not found", "Cannot add resource", "Resource not found", "Image not found", "Image memory error", "Pen does not exist", "Config type invalid", "Config token not found", "Config parse error", "Config memory error", "Bad external code format", "Bad external code offset", "External code not present", "Null window", "Destroy window error", "Null menu", "Print aborted", "Bad print record", "Print driver error", "Windows error during printing", "Memory error during printing", "Print dialog error", "Generic print error", "Invalid device refnum", "Device not found", "Device parameter error", "Device unit error", "Cannot open device", "Device call aborted", "Generic error", "Cancelled by user", "Object ID too low", "Object ID too high", "Object not in heap", "Unknown heap", "Unknown object (invalid DefProc)", "Unknown object (DefProc not in table)", "Message out of range", "Invalid (null) method", "Unknown message", "Manager call not supported", "Bad address", "Network operation in progress", "Network operation timed out", "Connection is busy", "Network attribute not supported", "Network error", "Address in use", "System out of memory", "Connection aborted", "Connection refused", "Not connected", "Already connected", "Connection closed", "Initialization error (interapplication manager)", "Bad occurrence", "Wait on unbound occurrence handler", "Occurrence queue overflow", "Datalog type conflict", "Unused", "Unrecognized type (interapplication manager)", "Memory corrupt", "Failed to make temporary DLL", "Old CIN version", "Drag socket not found", "Failed to load drop-object", "Failed to register OLE object", "Failed to release OLE object", "Format specifier type mismatch", "Unknown format specifier", "Too few format specifiers", "Too many format specifiers", "Scan failed", "Newer CIN version", "Error converting to variant", "Runtime menu error", "Password tampered", "Variant attribute not found", "Incompatible variant data type", "Event data is not available", "Event Store is not present", "Occurrence is not found", "Event Queue is not created", "Event info is not available", "Refnum passed is NULL", "Error retrieving Class GUID", "Error retrieving CoClass GUID", "Error retrieving TypeLib GUID.", "Bad built application magic bytes.", "Specific driver is different from the specific driver associated with the Logical Name.", "There is no session opened to the class driver.", "Max Error", "MAX - Error with config objects", "MAX - Error loading configuration", "MAX - Group not supported"]
        # "Current State"
        # "Do not delete, rename, or modify this frame.\n(this is used to capture unhandled states and typos)"
        # "Handle mistyped state name (developer tool)"
        n52 = Format Into String(format string="Software Exception: Unhandled State \"%s\"." ("message"), error in=w127, w122) -> (resulting string=w130:string, error out=w129:errorcluster)  [unwired: 1 in]
        n53 = call <vilib>:"Error Cluster From Error Code.vi"("show call chain? (False)"=TRUE, "error in (no error)"=w129, "error message (\"\")"=w130, "error code (0)"=w131) -> ("error out"=w128:errorcluster)  [unwired: 5 in]
        n54 = call <vilib>:"Add State(s) to Queue__jki_lib_state_machine.vi"("State(s) in (\"\")"=w126) -> ("States Out"=w125:string)  [unwired: 14 in]
      }
      frame "Initialize Core Data" {
        # "Do not delete, rename, or modify this frame.\n(this is used to determine panel behavior on exit)"
        # "originally closed?"
        # "exe?"
        # "If panel starts closed or is an EXE, then close it when we exit"
        n55 = property class="VI"() -> ("Front Panel.Open"=w140:bool)  [unwired: 2 in, 2 out]
        n56 = property class="App"() -> ("App.Kind"=w139:T8)  [unwired: 2 in, 2 out]
        n57 = control-ref of="Current VI Reference"() -> (w133:refnum<vi>)
        n58 = Not(x=w140) -> (.not. x?=w137:bool)
        n59 = Equal?(x=w139, y=T8."Run Time System" ("Application:Kind")) -> (x = y?=w136:bool)
        n60 = Or(x=w137, y=w136) -> (x .or. y?=w134:bool)
        n61 = Bundle By Name(cluster=w135, "Core.Current VI Reference"=w133, "Core.Close Panel on Exit?"=w134) -> (w142:T18)
        n62 = call <vilib>:"Add State(s) to Queue__jki_lib_state_machine.vi"("State(s) in (\"\")"=w144) -> ("States Out"=w143:string)  [unwired: 14 in]
      }
      frame "Error Handler" {
        # "Unhandled Error -- Display it"
        # "Handle any errors here.\nYou can also output any states to clean-up after errors occur"
        # "Clear error"
        n63 = call <vilib>:"General Error Handler.vi"("error in (no error)"=w146) -> ()  [unwired: 10 in, 5 out]
        n64 = call <vilib>:"Add State(s) to Queue__jki_lib_state_machine.vi"("State(s) in Front (\"\")"="/* Post Error States", "State(s) in (\"\")"=w150) -> ("States Out"=w149:string)  [unwired: 13 in]
      }
      frame "Exit" {
        # "Do not put any code in this frame.\n(No errors that occur here will be handled.)"
        n65 = call <vilib>:"Add State(s) to Queue__jki_lib_state_machine.vi"("State(s) in (\"\")"=w155) -> ("States Out"=w154:string)  [unwired: 14 in]
      }
      frame "---------- Data ----------" {
        # "Do not put any code in this frame.\n(It is a separator no-op. You can make a copy of this frame to create a new Data frame)"
        n66 = call <vilib>:"Add State(s) to Queue__jki_lib_state_machine.vi"("State(s) in (\"\")"=w159) -> ("States Out"=w158:string)  [unwired: 14 in]
      }
      frame "Data: Initialize" {
        w160 = ""  # comments
        w161 = T5."No Selection"  # KH ALL Buttons
        w162 = u16[] [] items=["", "I+", "I-", "V1+", "V1-", "V2+", "V2-", "V3+", "V3-", "V4+", "V4-", "Vsg", "Vbg", "user1", "user2"]  # Label
        w163 = ""  # device
        w164 = path ""  # path
        w165 = ""  # project
        w166 = ""  # user
        w167 = ""  # date
        w168 = ""  # canvas
        w169 = ""  # sample
        w170 = T4 [] items=["NC", "26", "27", "28", "1", "2", "3", "4", "5", "6", "7", "8", "9", "10", "11", "12", "13", "14", "15", "16", "17", "18", "19", "20", "21", "22", "23", "24", "25"]  # Electrode
        w171 = T2[] [] items=["Open", "50 Ohms", "500 Ohms", "5k Ohms", "50k Ohms"]  # Shunt Resistor
        w172 = enum16{"Ground", "Current", "Voltage", "Gate"}[] [enum."Current"] items=["Ground", "Current", "Voltage", "Gate"]  # Configuration
        w173 = T3[] [] items=["1x", "10x", "100x", "1000x"]  # Gain
        w174 = enum16{"1", "2", "3", "4", "5", "6", "7", "8"}[] [enum."1", enum."2", enum."3", enum."4", enum."5", enum."6", enum."7", enum."8"] items=["1", "2", "3", "4", "5", "6", "7", "8"]  # KH Ch
        w175 = enum16{"1", "2", "3", "4", "5", "6", "7", "8"}[] [enum."1", enum."2", enum."3", enum."4", enum."5", enum."6", enum."7", enum."8"] items=["1", "2", "3", "4", "5", "6", "7", "8"]  # Lockin Ch
        w176 = T15 [{"Channel"=enum."Channel 1", "Gain"=enum."1x", "Shunt Resistor"=enum."Open", "Input Config"=enum."Ground"}, {"Channel"=enum."Channel 2", "Gain"=enum."1x", "Shunt Resistor"=enum."Open", "Input Config"=enum."Ground"}, {"Channel"=enum."Channel 3", "Gain"=enum."1x", "Shunt Resistor"=enum."Open", "Input Config"=enum."Ground"}, {"Channel"=enum."Channel 4", "Gain"=enum."1x", "Shunt Resistor"=enum."Open", "Input Config"=enum."Ground"}, {"Channel"=enum."Channel 5", "Gain"=enum."1x", "Shunt Resistor"=enum."Open", "Input Config"=enum."Ground"}, {"Channel"=enum."Channel 6", "Gain"=enum."1x", "Shunt Resistor"=enum."Open", "Input Config"=enum."Ground"}, {"Channel"=enum."Channel 7", "Gain"=enum."1x", "Shunt Resistor"=enum."Open", "Input Config"=enum."Ground"}, {"Channel"=enum."Channel 8", "Gain"=enum."1x", "Shunt Resistor"=enum."Open", "Input Config"=enum."Ground"}]  # Channel Setting
        w177 = T19 {"Current VI Reference"=refnum, "Close Panel on Exit?"=FALSE}  # Core
        # "would probably be better as array of cluster of enums"
        # "Initialize the shift-register data, here.\n(data names are defined by what you wire into the bundle function)"
        n67 = Bundle("Core"=w177, "sample"=w169, "canvas"=w168, "date"=w167, "user"=w166, "project"=w165, "path"=w164, "device"=w163, "Channel Setting"=w176, "KH ALL Buttons"=w161, "Lockin Ch"=w175, "KH Ch"=w174, "Gain"=w173, "Configuration"=w172, "Shunt Resistor"=w171, "Electrode"=w170, "Label"=w162, "comments"=w160) -> (w179:T18)  [unwired: 1 in]
        n68 = call <vilib>:"Add State(s) to Queue__jki_lib_state_machine.vi"("State(s) in (\"\")"=w181) -> ("States Out"=w180:string)  [unwired: 14 in]
      }
      frame "Data: Cleanup" {
        # "Cleanup any data and references, here.\n(this is called automatically, by the Macro: Exit)"
        n69 = Unbundle By Name(w182) -> ("Core.Current VI Reference"=w185:refnum<vi>)
        n70 = Close Reference(reference=w185, error in (no error)=w184) -> (error out=w183:errorcluster)
        n71 = call <vilib>:"Add State(s) to Queue__jki_lib_state_machine.vi"("State(s) in (\"\")"=w187) -> ("States Out"=w186:string)  [unwired: 14 in]
      }
      frame "---------- UI ----------" {
        # "Do not put any code in this frame.\n(It is a separator no-op. You can make a copy of this frame to create a new UI frame)"
        n72 = call <vilib>:"Add State(s) to Queue__jki_lib_state_machine.vi"("State(s) in (\"\")"=w191) -> ("States Out"=w190:string)  [unwired: 14 in]
      }
      frame "UI: Initialize" {
        # "Initialize the User Interface, here.\n(this is called automatically, by the Macro: Init)"
        n73 = call <userlib>:"Fit VI window to Largest Dec__ogtk.vi"("error in (no error)"=w198) -> ("error out"=w192:errorcluster)  [unwired: 5 in, 1 out]
        n74 = local read "Pickering Buttons"() -> (w195:enum32{"Pickering", "Not Pickering"})
        n75 = local write "KH ALL Buttons"(T5."No Selection" ("Radio Buttons")) -> ()
        n76 = property on="Ring" class="Ring (strict)"(error in=w192, "Strings []"=string[] ["", "I+", "I-", "V1+", "V1-", "V2+", "V2-", "V3+", "V3-", "V4+", "V4-", "Vsg", "Vbg"] ("Strings [] 2")) -> (error out=w196:errorcluster)  [unwired: 1 in, 1 out]
        n77 = property on="Pickering Buttons" class="RadioBtnsControl (strict)"(error in=w196, "Val(Sgnl)"=w195) -> (error out=w194:errorcluster)  [unwired: 1 in, 1 out]
        n78 = call <vilib>:"Add State(s) to Queue__jki_lib_state_machine.vi"("State(s) in (\"\")"=w201) -> ("States Out"=w200:string)  [unwired: 14 in]
      }
      frame "UI: Cursor Set" {
        # "Argument"
        # "Set and Unset Cursor Busy.\n(Usage: \"UI: Cursor Set >> Busy|Idle\")"
        n79 = case shown="\"Idle\", Default" w202 {
          tunnel: w204 -> [w209 w211]
          tunnel: [w208 w210] -> w203
          frame "Idle", Default {
            n80 = call <vilib>:"Unset Busy.vi"("error in (no error)"=w209) -> ("error out"=w208:errorcluster)  [unwired: 10 in]
          }
          frame "Busy" {
            n81 = call <vilib>:"Set Busy.vi"("error in (no error)"=w211) -> ("error out"=w210:errorcluster)  [unwired: 9 in, 1 out]
          }
        }
        n82 = call <vilib>:"Add State(s) to Queue__jki_lib_state_machine.vi"("State(s) in (\"\")"=w207) -> ("States Out"=w206:string)  [unwired: 14 in]
      }
      frame "UI: Front Panel State" {
        # "Argument"
        # "Set Front Panel Open or Closed\n(Usage: \"UI: Front Panel State >> Open|Close\")"
        n83 = Unbundle By Name(w214) -> ("Core.Current VI Reference"=w213:refnum<vi>)
        n84 = case shown="\"Open\", Default" w212 {
          tunnel: w216 -> [w222 w235]
          tunnel: [w224 w236] -> w215
          tunnel: w213 -> [w223 w233]
          frame "Open", Default {
            n85 = property class="VI"(reference=w223, error in=w222) -> (reference out=w220:refnum<vi>, error out=w221:errorcluster, "Front Panel.Open"=w219:bool)
            n86 = case shown="False" w219 {
              tunnel: [w227 w230] -> w224
              tunnel: w221 -> [w226 w230]
              tunnel: w220 -> [w225 _]
              frame False {
                n87 = invoke class="VI" method="FP.Open"(reference=w225, error in=w226, "Activate"=TRUE, "State"=T9."Standard") -> (error out=w227:errorcluster)  [unwired: 1 in, 4 out]
              }
              frame True {
              }
            }
          }
          frame "Close" {
            n88 = property class="VI"(reference=w233, error in=w235) -> (reference out=w232:refnum<vi>, error out=w234:errorcluster, "Front Panel.Open"=w231:bool)
            n89 = case shown="True" w231 {
              tunnel: [w237 w240] -> w236
              tunnel: w234 -> [w237 w239]
              tunnel: w232 -> [_ w238]
              frame False {
              }
              frame True {
                n90 = invoke class="VI" method="FP.Close"(reference=w238, error in=w239) -> (error out=w240:errorcluster)  [unwired: 1 in, 2 out]
              }
            }
          }
        }
        n91 = call <vilib>:"Add State(s) to Queue__jki_lib_state_machine.vi"("State(s) in (\"\")"=w218) -> ("States Out"=w217:string)  [unwired: 14 in]
      }
      frame "---------- Macro ----------" {
        # "Do not put any code in this frame.\n(It is a separator no-op. You can make a copy of this frame to create a new Macro frame)"
        n92 = call <vilib>:"Add State(s) to Queue__jki_lib_state_machine.vi"("State(s) in (\"\")"=w244) -> ("States Out"=w243:string)  [unwired: 14 in]
      }
      frame "Macro: Initialize" {
        w245 = "Data: Initialize\nInitialize Core Data\nUI: Initialize\nUI: Front Panel State >> Open"  # Data: Initialize Initialize Core Data UI: Initialize UI: Front Panel State >> Open
        # "Initialization Macro\n(This is called once, when the VI starts)"
        n93 = call <vilib>:"Add State(s) to Queue__jki_lib_state_machine.vi"("State(s) in Front (\"\")"=w245, "State(s) in (\"\")"=w249) -> ("States Out"=w248:string)  [unwired: 13 in]
      }
      frame "Macro: Exit" {
        # "Exit Macro\n(This is called once, when the VI exits)"
        n94 = Unbundle By Name(w256) -> ("Core.Close Panel on Exit?"=w255:bool)
        n95 = Select(t="UI: Front Panel State >> Close", s=w255, f="") -> (s? t:f=w252:string)
        n96 = call <vilib>:"Add State(s) to Queue__jki_lib_state_machine.vi"("State(s) in (\"\")"=w252, "State(s) at Back (\"\")"="Data: Cleanup\nExit") -> ("States Out"=w250:string)  [unwired: 13 in]
        n97 = call <vilib>:"Add State(s) to Queue__jki_lib_state_machine.vi"("State(s) in Front (\"\")"=w250, "State(s) in (\"\")"=w259) -> ("States Out"=w258:string)  [unwired: 13 in]
      }
      frame "Macro: Output" {
        n98 = local read "Pickering Buttons"() -> (w264:enum32{"Pickering", "Not Pickering"})
        n99 = case shown="\"Pickering\", Default" w264 {
          tunnel: ["metadata: set Pickering" ("State(s) in Front (\"\")") "metadata: set KH" ("State(s) in Front (\"\")")] -> w262
          frame "Pickering", Default {
          }
          frame "Not Pickering" {
          }
        }
        n100 = call <vilib>:"Add State(s) to Queue__jki_lib_state_machine.vi"("State(s) in Front (\"\")"="metadata: update cluster\nmetadata: build path" ("State(s) in Front (\"\")"), "State(s) in (\"\")"=w262, "State(s) at Back (\"\")"="metadata: format comments\nmetadata: update globals\nmetadata: update fgv\nmetadata: create JSON" ("State(s) in Front (\"\")")) -> ("States Out"=w260:string)  [unwired: 12 in]
        n101 = call <vilib>:"Add State(s) to Queue__jki_lib_state_machine.vi"("State(s) in Front (\"\")"=w260, "State(s) in (\"\")"=w268) -> ("States Out"=w267:string)  [unwired: 13 in]
      }
      frame "---------- metadata ----------" {
        n102 = call <vilib>:"Add State(s) to Queue__jki_lib_state_machine.vi"("State(s) in (\"\")"=w274) -> ("States Out"=w273:string)  [unwired: 14 in]
      }
      frame "metadata: update cluster" {
        w288 = T15 [{"Channel"=enum."Channel 1", "Gain"=enum."1x", "Shunt Resistor"=enum."Open", "Input Config"=enum."Ground"}, {"Channel"=enum."Channel 2", "Gain"=enum."1x", "Shunt Resistor"=enum."Open", "Input Config"=enum."Ground"}, {"Channel"=enum."Channel 3", "Gain"=enum."1x", "Shunt Resistor"=enum."Open", "Input Config"=enum."Ground"}, {"Channel"=enum."Channel 4", "Gain"=enum."1x", "Shunt Resistor"=enum."Open", "Input Config"=enum."Ground"}, {"Channel"=enum."Channel 5", "Gain"=enum."1x", "Shunt Resistor"=enum."Open", "Input Config"=enum."Ground"}, {"Channel"=enum."Channel 6", "Gain"=enum."1x", "Shunt Resistor"=enum."Open", "Input Config"=enum."Ground"}, {"Channel"=enum."Channel 7", "Gain"=enum."1x", "Shunt Resistor"=enum."Open", "Input Config"=enum."Ground"}, {"Channel"=enum."Channel 8", "Gain"=enum."1x", "Shunt Resistor"=enum."Open", "Input Config"=enum."Ground"}]  # Channel Setting
        n103 = Bundle By Name(cluster=w290, "KH ALL Buttons"="KH ALL Buttons", "Channel Setting"=w288, "Lockin Ch"="Lockin Ch", "KH Ch"="KH Ch", "Gain"="KH Gain", "Configuration"="KH Configuration", "Shunt Resistor"="KH Shunt Resistor", "Electrode"="Electrode", "Label"="Label", "sample"="sample", "canvas"="canvas", "date"="device 2", "user"="user (emum?)", "project"="project (enum?)") -> (w289:T18)
        n104 = call <vilib>:"Add State(s) to Queue__jki_lib_state_machine.vi"("State(s) in (\"\")"=w293) -> ("States Out"=w292:string)  [unwired: 14 in]
      }
      frame "metadata: set KH" {
        n105 = Unbundle By Name(w301) -> ("Channel Setting"=w308:T15, "KH Ch"=w299:enum16{"1", "2", "3", "4", "5", "6", "7", "8"}[], "Gain"=w307:T3[], "Configuration"=w306:enum16{"Ground", "Current", "Voltage", "Gate"}[], "Shunt Resistor"=w305:T2[], "KH ALL Buttons"=w295:T5)
        n106 = local read "KH Configuration"() -> (w297:enum16{"Ground", "Current", "Voltage", "Gate"}[])
        n107 = for {
          tunnel: w308 -> [w326] mode=indexing
          tunnel: w306 -> [w327] mode=indexing
          tunnel: [w324] -> w309 mode=indexing
          tunnel: w307 -> [w323] mode=indexing
          tunnel: w305 -> [w321] mode=indexing
          tunnel: w299 -> [w320] mode=indexing
          tunnel: [w318] -> w294 mode=indexing
          n108 = case shown="\"Gate\"" w327 {
            tunnel: [Input_Configuration-Enum."Ground" ("Input Config") Input_Configuration-Enum."Differential" ("Input Config") Input_Configuration-Enum."SE+ (-gnd)" ("Input Config") Input_Configuration-Enum."Differential" ("Input Config")] -> w325
            tunnel: [Shunt-Enum."Open" ("Shunt Resistor") w331 Shunt-Enum."Open" ("Shunt Resistor") Shunt-Enum."50k Ohms" ("Shunt Resistor")] -> w318
            tunnel: w323 -> [_ w332 w335 w338]
            tunnel: [Gain-Enum."1x" ("Gain") w332 w335 w338] -> w322
            tunnel: w321 -> [_ w331 _ _]
            frame "Ground", Default {
            }
            frame "Current" {
            }
            frame "Voltage" {
            }
            frame "Gate" {
            }
          }
          n109 = To Unsigned Long Integer(number=w320) -> (unsigned 32bit integer=w319:u32)
          n110 = Bundle By Name(cluster=w326, "Channel"=w319, "Gain"=w322, "Input Config"=w325, "Shunt Resistor"=w318) -> (w324:T16)
        }
        n111 = for {
          tunnel: w295 -> [w314]
          tunnel: w297 -> [w313] mode=indexing
          tunnel: [w312] -> w296 mode=indexing
          n112 = case shown="\"all ground\"" w314 {
            tunnel: w313 -> [w315 _ _]
            tunnel: [w315 enum16{"Ground", "Current", "Voltage", "Gate"}."Ground" ("Enum 2") enum16{"Ground", "Current", "Voltage", "Gate"}."Current" ("Enum 2")] -> w312
            frame "No Selection", Default {
            }
            frame "all ground" {
            }
            frame "all differential" {
            }
          }
        }
        n113 = local write "KH ALL Buttons"(T5."No Selection" ("Radio Buttons")) -> ()
        n114 = local write "KH Configuration"(w296) -> ()
        n115 = call <userlib>:"KH Control.vi"("Radio Buttons"=w295, "error in"=w304, "Channel Setting"=w309) -> ("error out"=w303:errorcluster, "Channel Settings Used"=w302:T16[])  [unwired: 7 in]
        n116 = Bundle By Name(cluster=w301, "Channel Setting"=w302, "Shunt Resistor"=w294) -> (w300:T18)
        n117 = call <vilib>:"Add State(s) to Queue__jki_lib_state_machine.vi"("State(s) in (\"\")"=w311) -> ("States Out"=w310:string)  [unwired: 14 in]
      }
      frame "metadata: set Pickering" {
        # "Electrodes control chooses Y channels\nLabels control chooses Y channels"
        n118 = Unbundle By Name(w347) -> ("Electrode"=w345:T4, "Label"=w344:u16[])
        n119 = call "ElectrodesLabelsToPickeringChannels.vi"("error in (no error)"=w343, "Labels"=w344, "Electrodes"=w345) -> ("error out"=w342:errorcluster, "Y Channel Array"=w341:string[][], "X Channel Array"=w340:string[])  [unwired: 6 in]
        "X Channel Array" <- w340
        "Y Channel Array" <- w341
        n120 = disable-structure shown="Disabled" {
          disable-tunnel: [w353 _] -> w346
          disable-tunnel: w342 -> [w352 _]
          disable-tunnel: w341 -> [w351 _]
          disable-tunnel: w340 -> [w350 _]
          frame Disabled {
            n121 = call "Pickering 4 wire.vi"("error in (no error)"=w352, "Y Channels"=w351, "X Channels"=w350) -> ("error out"=w353:errorcluster)  [unwired: 7 in, 1 out]
          }
          frame Enabled {
          }
        }
        n122 = call <vilib>:"Add State(s) to Queue__jki_lib_state_machine.vi"("State(s) in (\"\")"=w349) -> ("States Out"=w348:string)  [unwired: 14 in]
      }
      frame "metadata: Pickering config" {
        n123 = case shown="\"Write\", Default" w354 {
          tunnel: w356 -> [w367 w372]
          tunnel: [w366 w371] -> w355
          frame "Write", Default {
            n124 = Bundle By Name(cluster=T11 {"x config"={"Electrode"=[], "X Channels"=[]}, "y config"={"Label"=[], "Y Channels"=[]}} ("Pickering Config"), "x config.Electrode"="Electrodes", "x config.X Channels"="X Channels", "y config.Label"="Labels", "y config.Y Channels"="Y Channels") -> (w365:T11)
            n125 = call "WritePickeringConfig.vi"("error in (no error)"=w367, "Pickering Config"=w365) -> ("Error Out"=w366:errorcluster)  [unwired: 9 in]
          }
          frame "Read" {
            n126 = call "ReadPickeringConfig.vi"("error in (no error)"=w372) -> ("error out"=w371:errorcluster, "Pickering Config"=w370:T11)  [unwired: 9 in]
            n127 = Unbundle By Name(w370) -> ("x config.Electrode"=w369:T4, "y config.Label"=w368:u16[])  [unwired: 2 out]
            n128 = local write "Electrodes"(w369) -> ()
            n129 = local write "Labels"(w368) -> ()
          }
        }
        n130 = call <vilib>:"Add State(s) to Queue__jki_lib_state_machine.vi"("State(s) in (\"\")"=w359) -> ("States Out"=w358:string)  [unwired: 14 in]
      }
      frame "metadata: build path" {
        n131 = Unbundle By Name(w382) -> ("project"=w376:string, "sample"=w375:string, "canvas"=w374:string, "date"=w384:string)
        n132 = Concatenate Strings(w375, w374, "." ("string"), w384) -> (w377:string)
        "device" <- w377
        "filename" <- w377
        n133 = Build Path(base path=path "G:/Team Drives/LevyLabData", name or relative path=w376) -> (appended path=w379:path)
        n134 = Build Path(base path=w379, name or relative path=w377) -> (appended path=w378:path)
        n135 = Path To String(path=w378) -> (string=→"folder":string)
        n136 = Bundle By Name(cluster=w382, "path"=w378, "device"=w377) -> (w381:T18)
        n137 = call <vilib>:"Add State(s) to Queue__jki_lib_state_machine.vi"("State(s) in (\"\")"=w387) -> ("States Out"=w386:string)  [unwired: 14 in]
      }
      frame "metadata: update globals" {
        n138 = Unbundle By Name(w390) -> ("path"=w392:path, "device"=w391:string)
        n139 = Unbundle By Name(w390) -> ("Label"=w389:u16[])  [unwired: 1 out]
        n140 = flat-sequence {
          tunnel: w389 -> [w402]
          tunnel: [w400] -> w388
          frame #0 {
            # "Code that searches for each label and outputs corresponding lockin channel"
            n141 = for {
              tunnel: w402 -> [w416] mode=indexing
              tunnel: [w417] -> w401 mode=indexing
              n142 = property on="Ring" class="Ring (strict)"() -> ("Strings []"=w418:string[])  [unwired: 2 in, 2 out]
              n143 = Index Array(array=w418, index=w416) -> (element=w417:string)
            }
            n144 = property on="Ring" class="Ring (strict)"() -> ("Strings []"=w396:string[])  [unwired: 2 in, 2 out]
            n145 = Array Size(array=w396) -> (size(s)=w399:i32)
            n146 = Initialize Array(-1 ("f"), w399) -> (w397:i32[])
            n147 = for {
              shift-right: [w409] -> w400
              shift-left: w397 -> [w410]
              tunnel: w396 -> [w406]
              tunnel: w401 -> [w407] mode=indexing
              i -> [w404]
              n148 = call <userlib>:"MGI Search Sorted.vi"("Search String"=w407, "Sorted Strings"=w406) -> ("Found"=w405:bool, "Closest Match"=w403:i32)  [unwired: 6 in, 2 out]
              n149 = case shown="True" w405 {
                tunnel: w410 -> [w411 w415]
                tunnel: [w411 w414] -> w409
                tunnel: w403 -> [_ w413]
                tunnel: w404 -> [_ w412]
                frame False {
                }
                frame True {
                  n150 = Replace Array Subset(array=w415, new element=w412, index=w413) -> (w414:i32[])
                }
              }
              n151 = Wait (ms)(milliseconds to wait=u32 0) -> ()  [unwired: 1 out]
            }
          }
        }
        n152 = flat-sequence {
          tunnel: w391 -> [w431]
          tunnel: w392 -> [w432]
          frame #0 {
            # "Existing: ITX Global"
            n153 = global write "ITX_Global.vi" "path"(w432) -> ()
            n154 = global write "ITX_Global.vi" "filename"(w431) -> ()
          }
        }
        n155 = flat-sequence {
          tunnel: w388 -> [w419]
          frame #0 {
            # "Existing: Channel Global"
            n156 = Index Array(array=w419) -> (element #2=w430:i32, element #3=w429:i32, element #4=w428:i32, element #5=w427:i32, element #6=w426:i32, element #7=w420:i32, element #8=w421:i32, element #9=w422:i32, element #10=w423:i32, element #11=w424:i32, element #12=w425:i32)  [unwired: 12 in, 1 out]
            n157 = global write "Channel Global.vi" "I+"(w430) -> ()
            n158 = global write "Channel Global.vi" "I-"(w429) -> ()
            n159 = global write "Channel Global.vi" "V1+"(w428) -> ()
            n160 = global write "Channel Global.vi" "V1-"(w427) -> ()
            n161 = global write "Channel Global.vi" "V2+"(w426) -> ()
            n162 = global write "Channel Global.vi" "V2-"(w420) -> ()
            n163 = global write "Channel Global.vi" "V3+"(w421) -> ()
            n164 = global write "Channel Global.vi" "V3-"(w422) -> ()
            n165 = global write "Channel Global.vi" "V4+"(w423) -> ()
            n166 = global write "Channel Global.vi" "V4-"(w424) -> ()
            n167 = global write "Channel Global.vi" "Vsg1"(w425) -> ()
          }
        }
        n168 = call <vilib>:"Add State(s) to Queue__jki_lib_state_machine.vi"("State(s) in (\"\")"=w395) -> ("States Out"=w394:string)  [unwired: 14 in]
      }
      frame "metadata: update fgv" {
        n169 = Unbundle By Name(w449) -> ("path"=w448:path, "device"=w438:string, "user"=w441:string, "comments"=w440:string, "Lockin Ch"=w447:enum16{"1", "2", "3", "4", "5", "6", "7", "8"}[], "Electrode"=w439:T4, "Label"=w446:u16[], "KH Ch"=w445:enum16{"1", "2", "3", "4", "5", "6", "7", "8"}[], "Configuration"=w444:enum16{"Ground", "Current", "Voltage", "Gate"}[], "Gain"=w443:T3[], "Shunt Resistor"=w442:T2[])
        n170 = Bundle By Name(cluster=T14 {"path"=path "", "device"="", "user"="", "comments"="", "Lockin Ch"=[], "Electrode"=[], "Label"=[], "KH Ch"=[], "Configuration"=[], "Gain"=[], "Shunt Resistor"=[]} ("Cluster in"), "path"=w448, "device"=w438, "user"=w441, "comments"=w440, "Lockin Ch"=w447, "Electrode"=w439, "Label"=w446, "KH Ch"=w445, "Configuration"=w444, "Gain"=w443, "Shunt Resistor"=w442) -> (w433:T14)
        n171 = call "Control Experiment FGV.vi"("Function"=enum16{"read", "write"}."write", "error in (no error)"=w436, "Cluster in"=w433) -> ("error out"=w435:errorcluster)  [unwired: 7 in, 1 out]
        n172 = call <vilib>:"Add State(s) to Queue__jki_lib_state_machine.vi"("State(s) in (\"\")"=w451) -> ("States Out"=w450:string)  [unwired: 14 in]
      }
      frame "metadata: format comments" {
        n173 = Unbundle By Name(w453) -> ("device"=w459:string, "project"=w458:string, "user"=w457:string)
        n174 = Unbundle By Name(w453) -> ("Lockin Ch"=w467:enum16{"1", "2", "3", "4", "5", "6", "7", "8"}[], "KH Ch"=w466:enum16{"1", "2", "3", "4", "5", "6", "7", "8"}[], "Gain"=w465:T3[], "Configuration"=w464:enum16{"Ground", "Current", "Voltage", "Gate"}[], "Shunt Resistor"=w463:T2[], "Electrode"=w462:T4, "Label"=w461:u16[])
        n175 = Bundle("description"="description", "device"=w459, "project"=w458, "user"=w457, "Lockin Ch"=w467, "KH Ch"=w466, "Gain"=w465, "Configuration"=w464, "Shunt Resistor"=w463, "Electrode"=w462, "Label"=w461) -> (w454:T20)  [unwired: 1 in]
        n176 = control-ref of="Ring"() -> (w456:refnum<vi>)
        n177 = call "Generate Comments.vi"("Ring in"=w456, "Cluster"=w454, "error in (no error)"=w455) -> ("Comments"=w452:string, "error out"=w468:errorcluster)  [unwired: 15 in]
        "comments" <- w452
        n178 = Bundle By Name(cluster=w453, "comments"=w452) -> ()  [unwired: 1 out]
        n179 = call <vilib>:"Add State(s) to Queue__jki_lib_state_machine.vi"("State(s) in (\"\")"=w470) -> ("States Out"=w469:string)  [unwired: 14 in]
      }
      frame "metadata: create JSON" {
        n180 = Unbundle(w488) -> ("sample"=w487:string, "canvas"=w485:string, "date"=w484:string, "user"=w483:string, "project"=w482:string, "path"=w481:path, "device"=w480:string, "Channel Setting"=w479:T15, "KH ALL Buttons"=w478:T5, "Lockin Ch"=w477:enum16{"1", "2", "3", "4", "5", "6", "7", "8"}[], "KH Ch"=w476:enum16{"1", "2", "3", "4", "5", "6", "7", "8"}[], "Gain"=w475:T3[], "Configuration"=w474:enum16{"Ground", "Current", "Voltage", "Gate"}[], "Shunt Resistor"=w473:T2[], "Electrode"=w472:T4, "Label"=w471:u16[])  [unwired: 2 out]
        n181 = Bundle("sample"=w487, "canvas"=w485, "date"=w484, "user"=w483, "project"=w482, "path"=w481, "device"=w480, "Channel Setting"=w479, "KH ALL Buttons"=w478, "Lockin Ch"=w477, "KH Ch"=w476, "Gain"=w475, "Configuration"=w474, "Shunt Resistor"=w473, "Electrode"=w472, "Label"=w471) -> (w486:T21)  [unwired: 1 in]
        n182 = call <vilib>:"Flatten To JSON String.vi"("Enums As String (F)"=TRUE, "Multiline (T)"=TRUE, "error in (no error)"=w490, "Variant"=w486) -> ("error out"=w489:errorcluster, "JSON String"=→"JSON String":string)  [unwired: 6 in]
        n183 = call <vilib>:"Add State(s) to Queue__jki_lib_state_machine.vi"("State(s) in (\"\")"=w495) -> ("States Out"=w494:string)  [unwired: 14 in]
      }
    }
  }
